vi "Color Band Test.vi"() -> ()   [LabVIEW 2020, in "VolatusGUIElements.lvlib" / "GaugeIndicator.lvclass"]
uses:
  GaugeIndicator.lvclass
  GaugeIndicator.lvclass/GaugeIndicator.ctl
panel:
  out "Gauge":dbl(knob)=6.270798808114836 scale=0.0..10.0
  out "Color Band":picture
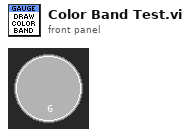
[diagram p1: front panel]
types:
  T1 = cluster{"Width":u16, "Style":enum32{"Solid", "Dash", "Dot", "DashDot", "DashDotDot"}}
  T2 = cluster{"left":i16, "top":i16, "right":i16, "bottom":i16}
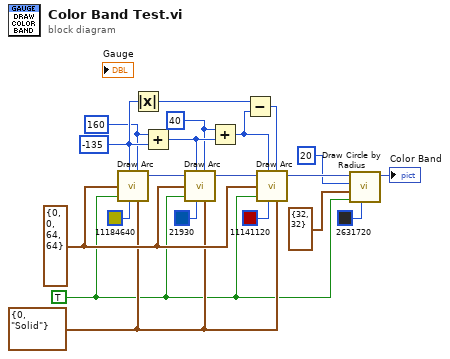
[diagram p0: block diagram]
diagram:
  w15 = i16 40 ("arc size[degrees]")
  w18 = i16 160 ("start angle[degrees]")
  w19 = i16 -135 ("start angle[degrees]")
  w11 = T1 {"Width"=0, "Style"=enum."Solid"} ("pen")
  w3 = TRUE ("fill?(F)")
  w13 = T2 {"left"=0, "top"=0, "right"=64, "bottom"=64} ("rect")
  n1 = call <vilib>:"Draw Arc.vi"("start angle[degrees]"=w19, "rect"=w13, "fill?(F)"=w3, "color(black)"=u32 11184640, "arc size[degrees]"=w18, "pen"=w11) -> ("new picture"=w17:picture)  [unwired: 3 in]
  n2 = Absolute Value(x=w19) -> (abs(x)=w8:i16)
  n3 = Add(x=w18, y=w19) -> (x+y=w16:i16)
  n4 = call <vilib>:"Draw Arc.vi"("picture"=w17, "start angle[degrees]"=w16, "rect"=w13, "fill?(F)"=w3, "color(black)"=u32 21930, "arc size[degrees]"=w15, "pen"=w11) -> ("new picture"=w10:picture)  [unwired: 2 in]
  n5 = Add(x=w15, y=w16) -> (x+y=w9:i16)
  n6 = Subtract(x=w8, y=w9) -> (x-y=w7:i16)
  n7 = call <vilib>:"Draw Arc.vi"("picture"=w10, "start angle[degrees]"=w9, "rect"=w13, "fill?(F)"=w3, "color(black)"=u32 11141120, "arc size[degrees]"=w7, "pen"=w11) -> ("new picture"=w6:picture)  [unwired: 2 in]
  n8 = call <vilib>:"Draw Circle by Radius.vi"("color(black)"=u32 2631720, "fill?(F)"=w3, "pixel center"=cluster{"horizontal":i16, "vertical":i16} {"horizontal"=32, "vertical"=32}, "radius"=i16 20, "picture"=w6) -> ("new picture"=→"Color Band":picture)  [unwired: 6 in]
